vi "IPS120 Control Panel.vi"(8 "error in (no error)":errorcluster, 11 "Class":refnum<class "IPS120.lvclass">) -> (0 "error out":errorcluster, 3 "IPS120 out":refnum<class "IPS120.lvclass">)   [LabVIEW 2015, in "IPS120.lvclass"]
uses:
  IPS120.lvclass
panel:
  in  "Data":cluster{"Channels to measure":i32[]}={"Channels to measure"=[8]}
  # "0: Demand current\n2: Measured current\n7: Demand field\n\nmore in manual pg.33"
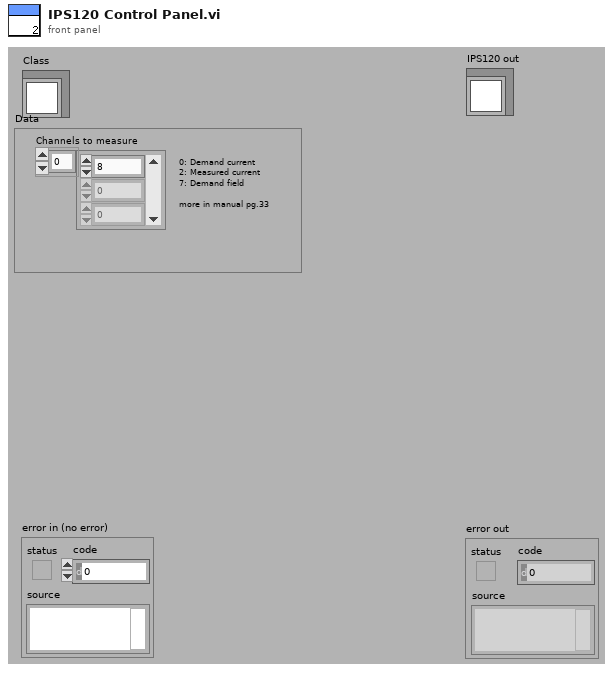
[diagram p1: front panel]
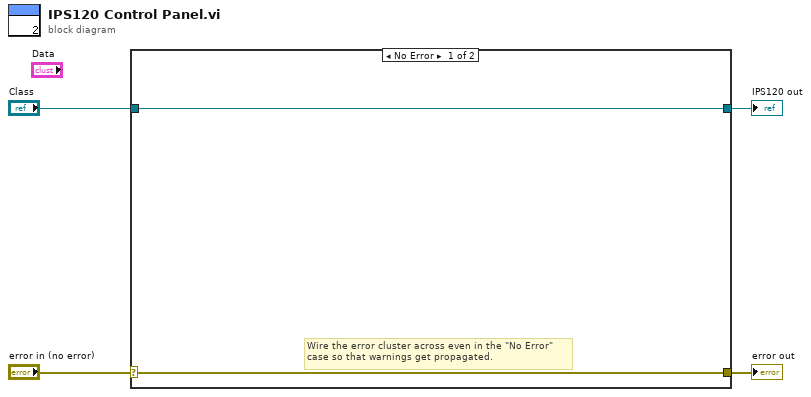
[diagram p0: block diagram]
diagram:
  n1 = case shown="No Error" "error in (no error)" {
    selector: "error in (no error)" -> [w5 w8]
    tunnel: [w5 w8] -> w3
    tunnel: [w6 w7] -> w1
    tunnel: "Class" -> [w6 w7]
    frame No Error {
      # "Wire the error cluster across even in the \"No Error\"\ncase so that warnings get propagated."
    }
    frame Error {
    }
  }
  "error out" <- w3
  "IPS120 out" <- w1
